vi "AutoWfmToSpreadsheet.vi"() -> ()   [LabVIEW 2017]
uses:
  <vilib>/Waveform/WDTFileIO.llb/Read Waveform from File.vi
  <vilib>/Waveform/WDTOps.llb/WDT Index Channel DBL.vi
  <vilib>/measure/maspectr.llb/FFT Power Spectrum and PSD for 1 Chan.vi
  <vilib>/Waveform/WDTFileIO.llb/Export Waveforms To Spreadsheet File (1D).vi
  <vilib>/measure/NI_MAPro.lvlib
panel:
  out "POWER":dbl[](graph)
  out "?":string
  out "Sinal adquirido":waveform(dbl)(graph)
  in  "?":bool
  in  "Escolher arquivo":i32
  out "Sinal de Referência":waveform(dbl)(graph)
  in  "V para Exportar/ F para Visualizar":bool
  out "result string":string
  in  "Local da pasta com arquivos wfm":path=path "C:/Users/lucas/Documents/GitHub/INT/Novo Ensaio US/NOVOS_SINAIS/sinais/wfm"
  out "element":string
  out "Numeric":i32
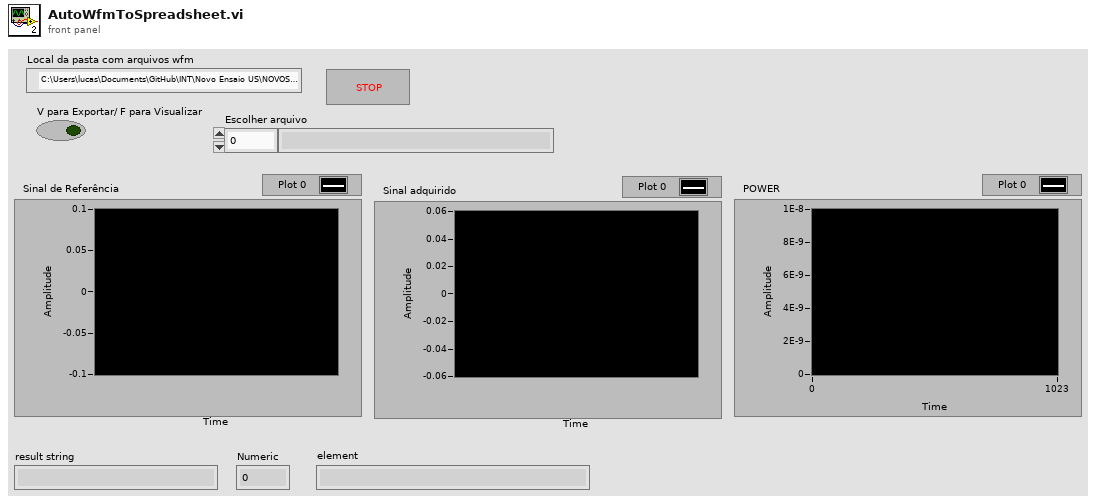
[diagram p1: front panel]
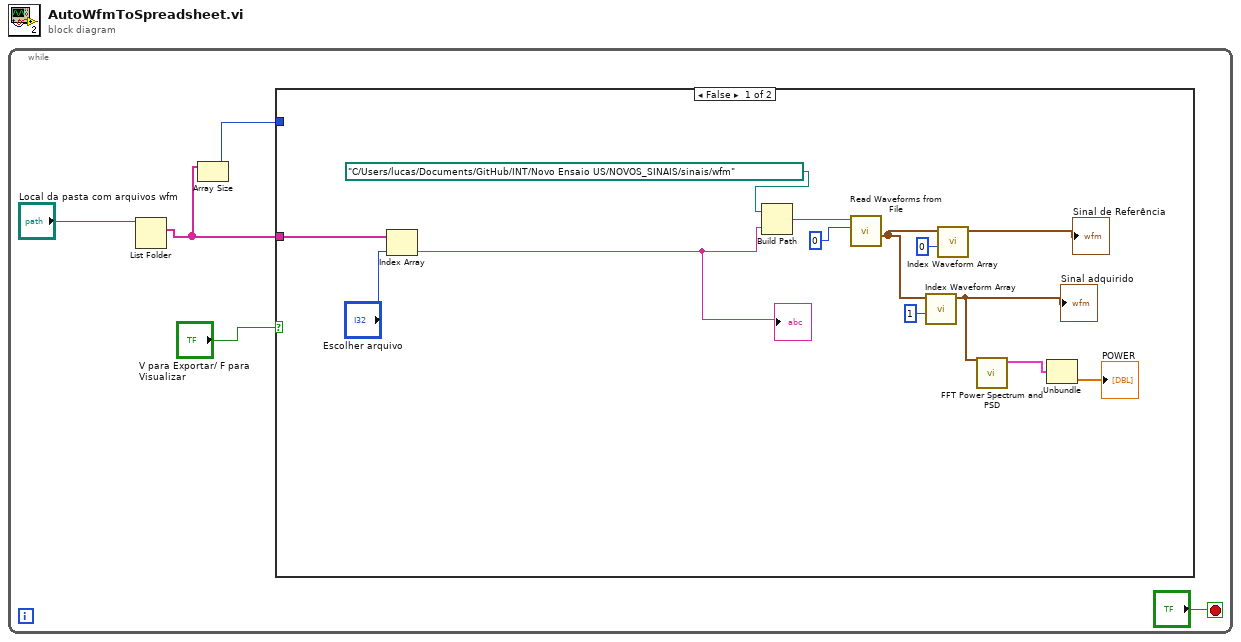
[diagram p0: block diagram]
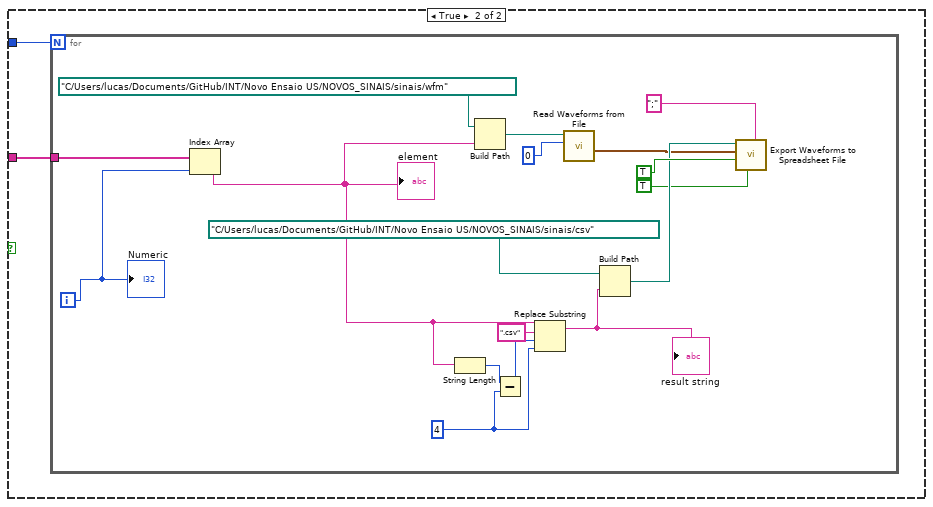
[diagram p2: hidden frame]
diagram:
  n1 = while {
    stop <- "?" stop-if-true
    n2 = List Folder(path="Local da pasta com arquivos wfm") -> (filenames=w4:string[])  [unwired: 3 in, 3 out]
    n3 = Array Size(array=w4) -> (size(s)=w3:i32)
    n4 = case shown="False" "V para Exportar/ F para Visualizar" {
      tunnel: w4 -> [w15 w20]
      tunnel: w3 -> [_ w19]
      frame False {
        n5 = Index Array(array=w15, index="Escolher arquivo") -> (element=w10:string)
        "?" <- w10
        n6 = Build Path(base path=path "C:/Users/lucas/Documents/GitHub/INT/Novo Ensaio US/NOVOS_SINAIS/sinais/wfm" ("file path (dialog if empty)"), name or relative path=w10) -> (appended path=w18:path)
        n7 = call-poly <vilib>:"Read Waveforms from File.vi"("offset (records:0)"=0, "file path (dialog if empty)"=w18) -> ("all waveforms in record"=w11:waveform(dbl)[])  [unwired: 4 in, 3 out]
        n8 = call-poly <vilib>:"Index Waveform Array.vi"("index"=1, "waveform array"=w11) -> ("waveform"=w6:waveform(dbl))  [unwired: 8 in, 1 out]
        "Sinal adquirido" <- w6
        n9 = call-poly <vilib>:"Index Waveform Array.vi"("index"=0, "waveform array"=w11) -> ("waveform"=→"Sinal de Referência":waveform(dbl))  [unwired: 8 in, 1 out]
        n10 = call-poly <vilib>:"FFT Power Spectrum and PSD.vi"("time signal"=w6) -> ("Power Spectrum / PSD"=w7:cluster{"f0":dbl, "df":dbl, "magnitude":dbl[]})  [unwired: 7 in, 3 out]
        n11 = Unbundle(w7) -> ("magnitude"=→"POWER":dbl[])  [unwired: 2 out]
      }
      frame True {
        n12 = for {
          N: w19 -> [_]
          tunnel: w20 -> [w37]
          i -> [w36]
          w24 = 4 ("length (len. of substring)")
          n13 = Index Array(array=w37, index=w36) -> (element=w25:string)
          "element" <- w25
          n14 = String Length(string=w25) -> (length=w23:i32)
          n15 = Build Path(base path=path "C:/Users/lucas/Documents/GitHub/INT/Novo Ensaio US/NOVOS_SINAIS/sinais/wfm" ("file path (dialog if empty)"), name or relative path=w25) -> (appended path=w33:path)
          n16 = Subtract(x=w23, y=w24) -> (x-y=w22:i32)
          n17 = Replace Substring(2:w24, 3:w22, 4:".csv" ("substring (\"\")"), 5:w25) -> (1:w26:string)  [unwired: 1 out]
          "result string" <- w26
          n18 = call-poly <vilib>:"Read Waveforms from File.vi"("offset (records:0)"=0, "file path (dialog if empty)"=w33) -> ("all waveforms in record"=w21:waveform(dbl)[])  [unwired: 4 in, 3 out]
          n19 = Build Path(base path=path "C:/Users/lucas/Documents/GitHub/INT/Novo Ensaio US/NOVOS_SINAIS/sinais/csv" ("file path (dialog if empty)"), name or relative path=w26) -> (appended path=w29:path)
          n20 = call-poly <vilib>:"Export Waveforms to Spreadsheet File.vi"("delimiter (Tab)"=";", "append to file? (new file:F)"=TRUE, "multiple time columns? (single:F)"=TRUE, "waveforms"=w21, "file path (dialog if empty)"=w29) -> ()  [unwired: 5 in, 2 out]
          "Numeric" <- w36
        }
      }
    }
  }
